vi "HTVacuum.ProcCases.vi"(0 "i ref in":refnum<vi>, 1 "selector":string, 2 "Data":T1, 3 "call cluster":T2={"Object"="", "Selector"="", "CallType"=enum."synchronous", "Async Object"="", "Async Selector"="", "Data Descriptor"="", "Data"=[], "Error #"=0, "Expire"=0}, 5 "error in (no error)":errorcluster) -> (14 "i ref out":refnum<vi>, 17 "answer cluster":T2={"Object"="", "Selector"="", "CallType"=enum."synchronous", "Async Object"="", "Async Selector"="", "Data Descriptor"="", "Data"=[], "Error #"=0, "Expire"=0}, 19 "error out":errorcluster)   [LabVIEW 2014, in "HTVacuum.lvlib"]
doc: "This method is called by a process from within the default case in the event loop. The methods of a class that are linked to events will be called from THIS method. Add your code here."
uses:
  HTVacuum.lvlib
  CS_Core/CSSystem/CoreDefs/CoreDefs.call_type.ctl
  CS_Core/BaseProcess/BaseProcess.descriptor string definition.ctl
  CS_Core/CSSystem/CoreDefs/CoreDefs.rawDataType.ctl
  CS_Core/CSSystem/CoreLib/CoreLib.string 2 byte array.vi
  CS_Core/CSSystem/CoreLib/CoreLib.short 2 byte array.vi
  CS_Core/CSSystem/CoreLib/CoreLib.byte array 2 int.vi
  CS_Core/CSSystem/CoreLib/CoreLib.int 2 byte array.vi
  CS_Core/BaseProcess/BaseProcess.lvlib
  CS_Core/CSSystem/CoreLib/CoreLib.lvlib
  CS_Core/CSApplicationBaseClasses/DeviceBase/DeviceBase.lvlib
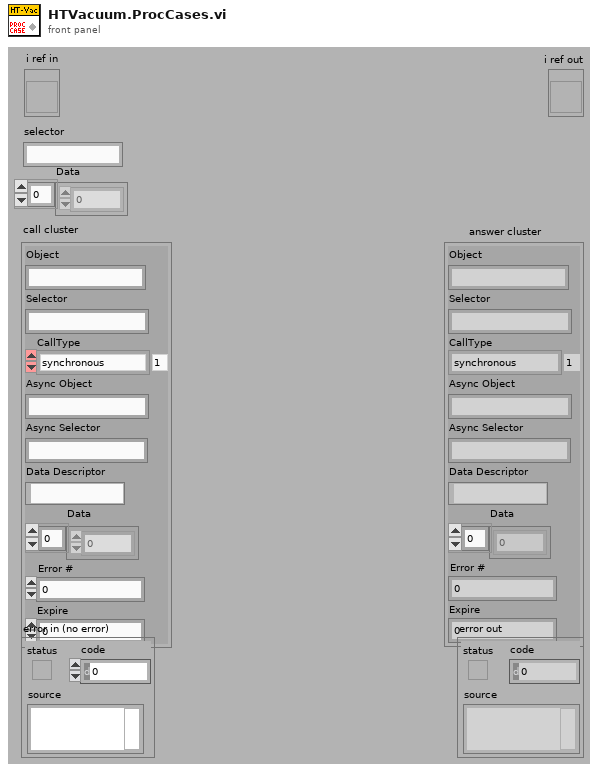
[diagram p1: front panel]
types:
  T1 = typedef "CoreDefs.rawDataType.ctl" = i8[]
  T2 = typedef "CoreDefs.call_type.ctl" = cluster{"Object":string, "Selector":string, "CallType":enum16{"simple", "synchronous", "asynchronous"}, "Async Object":string, "Async Selector":string, "Data Descriptor":T3, "Data":T1, "Error #":i32, "Expire":u32}
  T3 = typedef "BaseProcess.lvlib/BaseProcess.descriptor string definition.ctl" = string
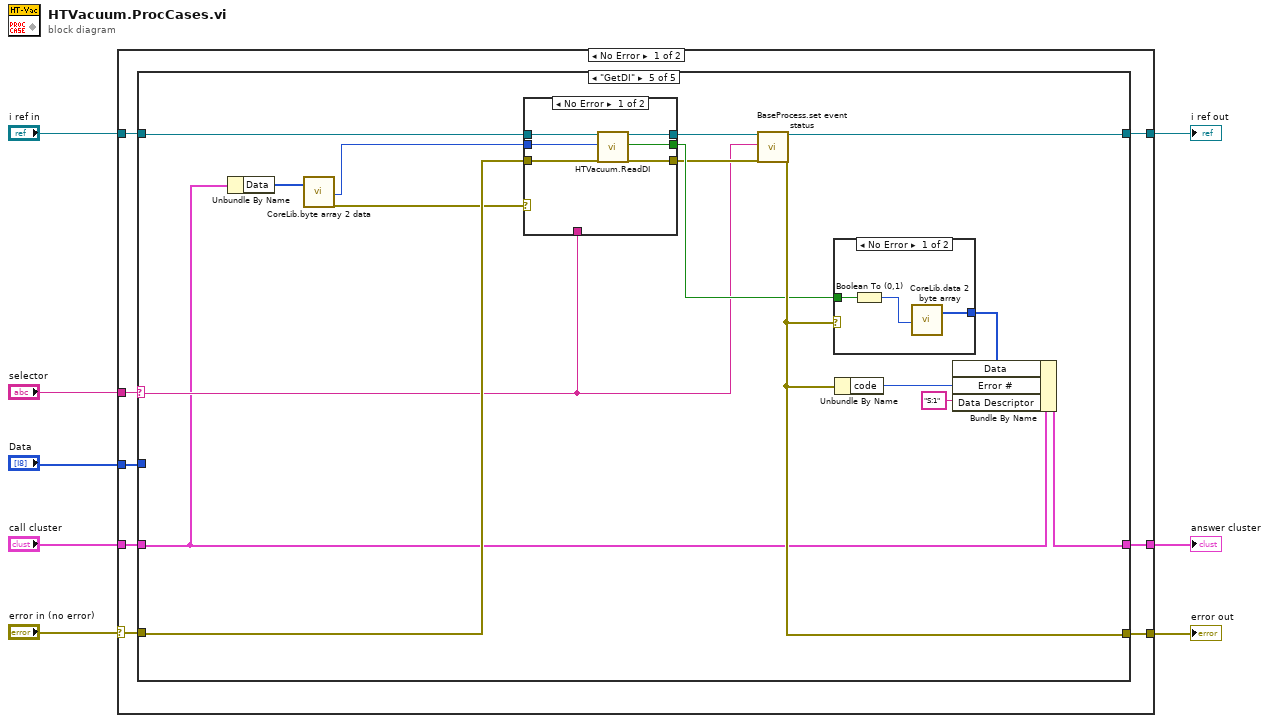
[diagram p0: block diagram]
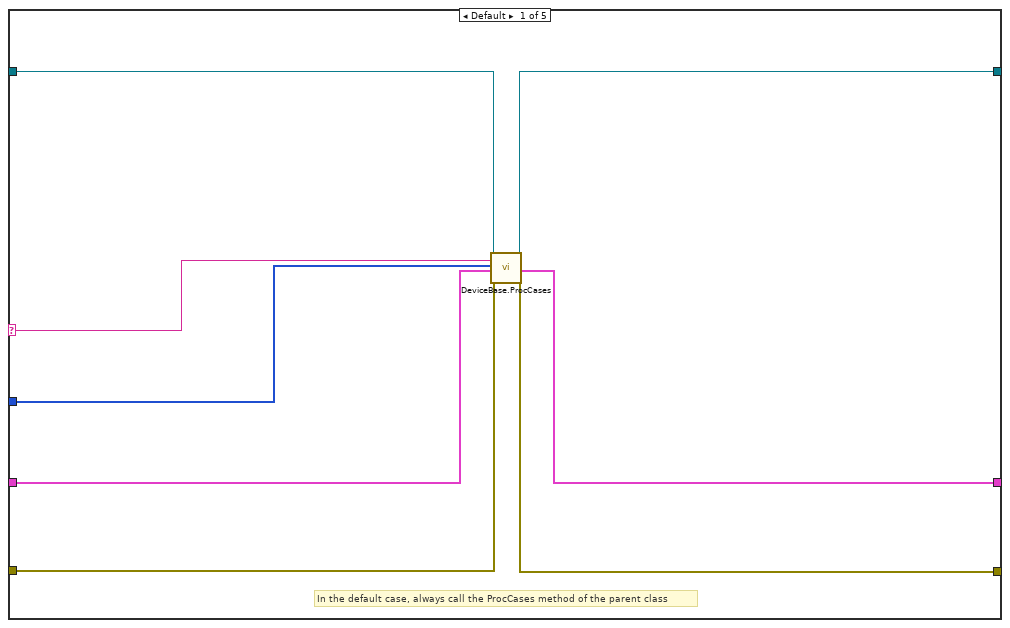
[diagram p2: hidden frame]
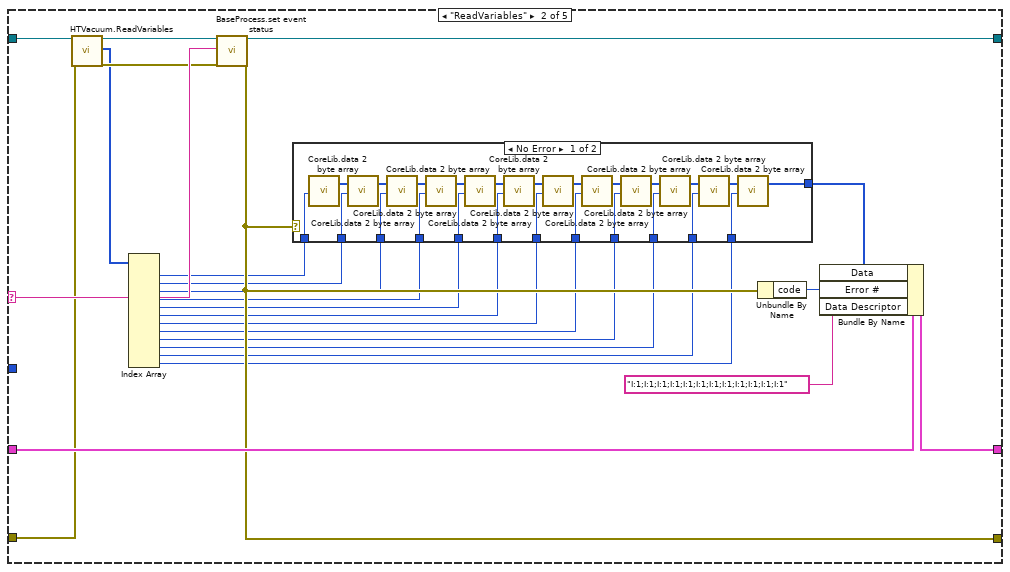
[diagram p3: hidden frame]
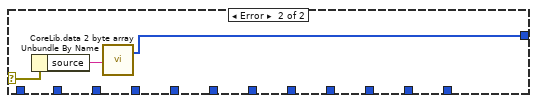
[diagram p4: hidden frame]
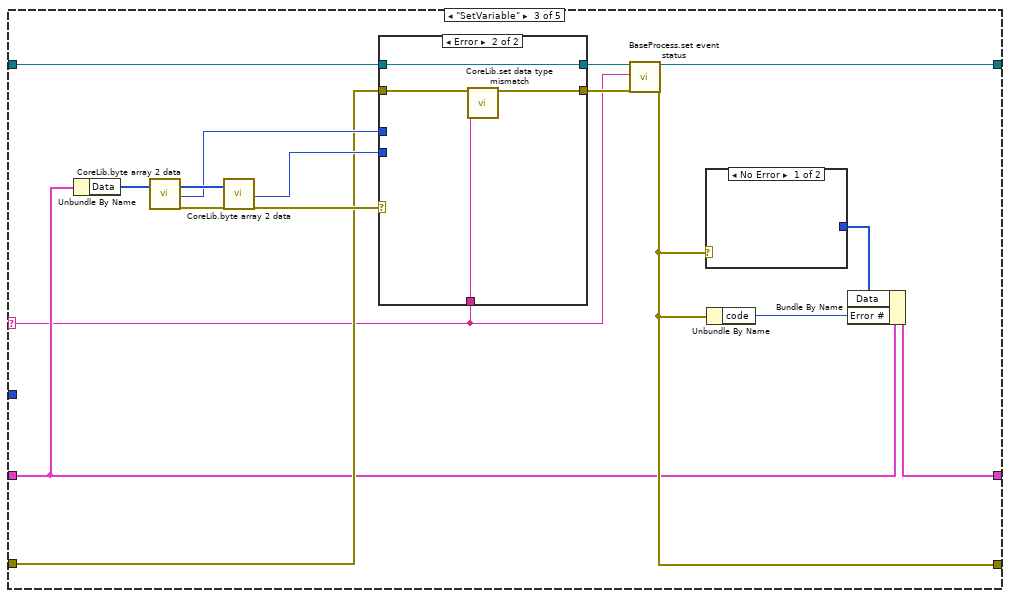
[diagram p5: hidden frame]
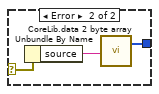
[diagram p6: hidden frame]
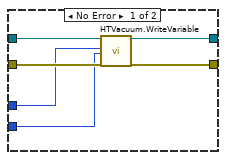
[diagram p7: hidden frame]
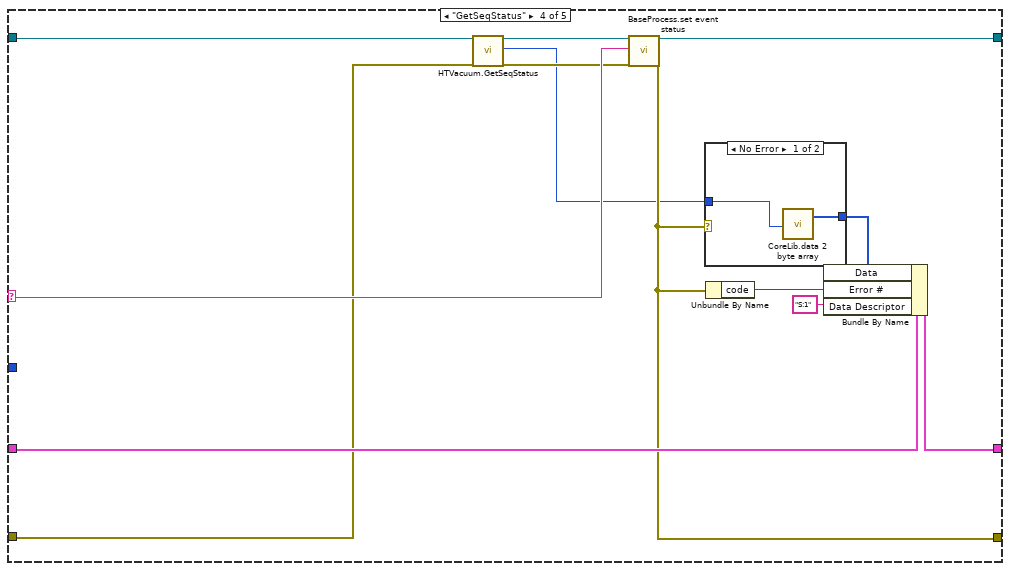
[diagram p8: hidden frame]
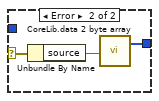
[diagram p9: hidden frame]
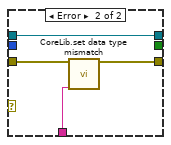
[diagram p10: hidden frame]
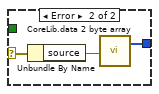
[diagram p11: hidden frame]
diagram:
  n1 = case shown="No Error" "error in (no error)" {
    selector: "error in (no error)" -> [w9 w157]
    tunnel: "selector" -> [w16 _]
    tunnel: [w15 w158] -> w7
    tunnel: "Data" -> [w14 _]
    tunnel: "call cluster" -> [w13 w158]
    tunnel: "i ref in" -> [w12 w159]
    tunnel: [w11 w159] -> w3
    tunnel: [w10 w157] -> w2
    frame No Error {
      n2 = case shown="\"GetDI\"" w16 {
        selector: w16 -> [w20 w44 w78 w115 w129]
        tunnel: w14 -> [w19 _ _ _ _]
        tunnel: w12 -> [w24 w41 w79 w111 w134]
        tunnel: [w23 w43 w77 w116 w137] -> w11
        tunnel: w13 -> [w18 w48 w80 w114 w126]
        tunnel: [w17 w47 w81 w113 w136] -> w15
        tunnel: w9 -> [w22 w38 w83 w109 w131]
        tunnel: [w21 w45 w82 w112 w135] -> w10
        frame Default {
          # "In the default case, always call the ProcCases method of the parent class"
          n3 = call "DeviceBase.ProcCases.vi"("i ref in"=w24, "selector"=w20, "Data"=w19, "call cluster"=w18, "error in (no error)"=w22) -> ("i ref out"=w23:refnum<vi>, "answer cluster"=w17:T2, "error out"=w21:errorcluster)  [unwired: 12 in]
        }
        frame "ReadVariables" {
          n4 = call "HTVacuum.ReadVariables.vi"("i ref in"=w41, "error in (no error)"=w38) -> ("i ref out"=w40:refnum<vi>, "U-VAR values"=w37:i32[], "error out"=w39:errorcluster)  [unwired: 15 in]
          n5 = Index Array(array=w37) -> (element #1=w36:i32, element #2=w35:i32, element #3=w34:i32, element #4=w33:i32, element #5=w32:i32, element #6=w31:i32, element #7=w30:i32, element #8=w29:i32, element #9=w28:i32, element #10=w27:i32, element #11=w26:i32, element #12=w25:i32)  [unwired: 12 in]
          n6 = call "BaseProcess.set event status.vi"("i ref in"=w40, "EventStatus"=w44, "error in (no error)"=w39) -> ("i ref out"=w43:refnum<vi>, "error out"=w45:errorcluster)  [unwired: 14 in, 1 out]
          n7 = case shown="No Error" w45 {
            selector: w45 -> [_ w76]
            tunnel: [w73 w75] -> w46
            tunnel: w36 -> [w61 _]
            tunnel: w35 -> [w60 _]
            tunnel: w34 -> [w59 _]
            tunnel: w33 -> [w58 _]
            tunnel: w32 -> [w57 _]
            tunnel: w31 -> [w56 _]
            tunnel: w30 -> [w55 _]
            tunnel: w29 -> [w54 _]
            tunnel: w28 -> [w53 _]
            tunnel: w27 -> [w52 _]
            tunnel: w26 -> [w51 _]
            tunnel: w25 -> [w50 _]
            frame No Error {
              n8 = call-poly "CoreLib.data 2 byte array.vi"("i32"=w61) -> ("byteArray out"=w62:T1)  [unwired: 18 in]
              n9 = call-poly "CoreLib.data 2 byte array.vi"("byteArray"=w62, "i32"=w60) -> ("byteArray out"=w63:T1)  [unwired: 17 in]
              n10 = call-poly "CoreLib.data 2 byte array.vi"("byteArray"=w63, "i32"=w59) -> ("byteArray out"=w64:T1)  [unwired: 17 in]
              n11 = call-poly "CoreLib.data 2 byte array.vi"("byteArray"=w64, "i32"=w58) -> ("byteArray out"=w65:T1)  [unwired: 17 in]
              n12 = call-poly "CoreLib.data 2 byte array.vi"("byteArray"=w65, "i32"=w57) -> ("byteArray out"=w66:T1)  [unwired: 17 in]
              n13 = call-poly "CoreLib.data 2 byte array.vi"("byteArray"=w66, "i32"=w56) -> ("byteArray out"=w67:T1)  [unwired: 17 in]
              n14 = call-poly "CoreLib.data 2 byte array.vi"("byteArray"=w67, "i32"=w55) -> ("byteArray out"=w68:T1)  [unwired: 17 in]
              n15 = call-poly "CoreLib.data 2 byte array.vi"("byteArray"=w68, "i32"=w54) -> ("byteArray out"=w69:T1)  [unwired: 17 in]
              n16 = call-poly "CoreLib.data 2 byte array.vi"("byteArray"=w69, "i32"=w53) -> ("byteArray out"=w70:T1)  [unwired: 17 in]
              n17 = call-poly "CoreLib.data 2 byte array.vi"("byteArray"=w70, "i32"=w52) -> ("byteArray out"=w71:T1)  [unwired: 17 in]
              n18 = call-poly "CoreLib.data 2 byte array.vi"("byteArray"=w71, "i32"=w51) -> ("byteArray out"=w72:T1)  [unwired: 17 in]
              n19 = call-poly "CoreLib.data 2 byte array.vi"("byteArray"=w72, "i32"=w50) -> ("byteArray out"=w73:T1)  [unwired: 17 in]
            }
            frame Error {
              n20 = Unbundle By Name(w76) -> ("source"=w74:string)
              n21 = call-poly "CoreLib.data 2 byte array.vi"("string"=w74) -> ("byteArray out"=w75:T1)  [unwired: 18 in]
            }
          }
          n22 = Unbundle By Name(w45) -> ("code"=w49:i32)
          n23 = Bundle By Name(cluster=w48, "Data"=w46, "Error #"=w49, "Data Descriptor"="I:1;I:1;I:1;I:1;I:1;I:1;I:1;I:1;I:1;I:1;I:1;I:1") -> (w47:T2)
        }
        frame "SetVariable" {
          n24 = Unbundle By Name(w80) -> ("Data"=w89:T1)
          n25 = call-poly "CoreLib.byte array 2 data.vi"("byteArray"=w89) -> ("byteArray out"=w87:T1, "i32"=w85:i32, "error out"=w88:errorcluster)  [unwired: 16 in]
          n26 = call-poly "CoreLib.byte array 2 data.vi"("byteArray"=w87, "error in (no error)"=w88) -> ("i32"=w84:i32, "error out"=w86:errorcluster)  [unwired: 15 in, 1 out]
          n27 = case shown="Error" w86 {
            tunnel: [w101 w106] -> w91
            tunnel: w79 -> [w102 w106]
            tunnel: w83 -> [w100 w105]
            tunnel: [w99 w104] -> w90
            tunnel: w84 -> [w98 _]
            tunnel: w78 -> [_ w103]
            tunnel: w85 -> [w97 _]
            frame No Error {
              n28 = call "HTVacuum.WriteVariable.vi"("i ref in"=w102, "Var# (1)"=w97, "Value"=w98, "error in (no error)"=w100) -> ("i ref out"=w101:refnum<vi>, "error out"=w99:errorcluster)  [unwired: 14 in]
            }
            frame Error {
              n29 = call "CoreLib.set data type mismatch.vi"("error in (no error)"=w105, "error source"=w103) -> ("error out"=w104:errorcluster)  [unwired: 17 in]
            }
          }
          n30 = call "BaseProcess.set event status.vi"("i ref in"=w91, "EventStatus"=w78, "error in (no error)"=w90) -> ("i ref out"=w77:refnum<vi>, "error out"=w82:errorcluster)  [unwired: 14 in, 1 out]
          n31 = case shown="No Error" w82 {
            selector: w82 -> [_ w96]
            tunnel: [_ w95] -> w92
            frame No Error {
            }
            frame Error {
              n32 = Unbundle By Name(w96) -> ("source"=w94:string)
              n33 = call-poly "CoreLib.data 2 byte array.vi"("string"=w94) -> ("byteArray out"=w95:T1)  [unwired: 18 in]
            }
          }
          n34 = Unbundle By Name(w82) -> ("code"=w93:i32)
          n35 = Bundle By Name(cluster=w80, "Data"=w92, "Error #"=w93) -> (w81:T2)
        }
        frame "GetSeqStatus" {
          n36 = call "HTVacuum.GetSeqStatus.vi"("i ref in"=w111, "error in (no error)"=w109) -> ("i ref out"=w110:refnum<vi>, "SeqStatus"=w107:u8, "error out"=w108:errorcluster)  [unwired: 15 in]
          n37 = call "BaseProcess.set event status.vi"("i ref in"=w110, "EventStatus"=w115, "error in (no error)"=w108) -> ("i ref out"=w116:refnum<vi>, "error out"=w112:errorcluster)  [unwired: 14 in, 1 out]
          n38 = case shown="No Error" w112 {
            selector: w112 -> [_ w124]
            tunnel: [w121 w122] -> w118
            tunnel: w107 -> [w120 _]
            frame No Error {
              n39 = call-poly "CoreLib.data 2 byte array.vi"("i16"=w120) -> ("byteArray out"=w121:T1)  [unwired: 18 in]
            }
            frame Error {
              n40 = Unbundle By Name(w124) -> ("source"=w123:string)
              n41 = call-poly "CoreLib.data 2 byte array.vi"("string"=w123) -> ("byteArray out"=w122:T1)  [unwired: 18 in]
            }
          }
          n42 = Unbundle By Name(w112) -> ("code"=w119:i32)
          n43 = Bundle By Name(cluster=w114, "Data"=w118, "Error #"=w119, "Data Descriptor"="S:1") -> (w113:T2)
        }
        frame "GetDI" {
          n44 = Unbundle By Name(w126) -> ("Data"=w128:T1)
          n45 = call-poly "CoreLib.byte array 2 data.vi"("byteArray"=w128) -> ("i32"=w125:i32, "error out"=w127:errorcluster)  [unwired: 16 in, 1 out]
          n46 = case shown="No Error" w127 {
            tunnel: w134 -> [w146 w147]
            tunnel: [w145 w147] -> w133
            tunnel: [w144 _] -> w132
            tunnel: w131 -> [w143 w150]
            tunnel: [w142 w149] -> w130
            tunnel: w129 -> [_ w148]
            tunnel: w125 -> [w141 _]
            frame No Error {
              n47 = call "HTVacuum.ReadDI.vi"("i ref in"=w146, "Port#"=w141, "error in (no error)"=w143) -> ("i ref out"=w145:refnum<vi>, "Port Status"=w144:bool, "error out"=w142:errorcluster)  [unwired: 14 in]
            }
            frame Error {
              n48 = call "CoreLib.set data type mismatch.vi"("error in (no error)"=w150, "error source"=w148) -> ("error out"=w149:errorcluster)  [unwired: 17 in]
            }
          }
          n49 = call "BaseProcess.set event status.vi"("i ref in"=w133, "EventStatus"=w129, "error in (no error)"=w130) -> ("i ref out"=w137:refnum<vi>, "error out"=w135:errorcluster)  [unwired: 14 in, 1 out]
          n50 = case shown="No Error" w135 {
            selector: w135 -> [_ w156]
            tunnel: [w153 w154] -> w139
            tunnel: w132 -> [w152 _]
            frame No Error {
              n51 = Boolean To (0,1)(Boolean=w152) -> (0, 1=w151:i16)
              n52 = call-poly "CoreLib.data 2 byte array.vi"("i16"=w151) -> ("byteArray out"=w153:T1)  [unwired: 18 in]
            }
            frame Error {
              n53 = Unbundle By Name(w156) -> ("source"=w155:string)
              n54 = call-poly "CoreLib.data 2 byte array.vi"("string"=w155) -> ("byteArray out"=w154:T1)  [unwired: 18 in]
            }
          }
          n55 = Unbundle By Name(w135) -> ("code"=w140:i32)
          n56 = Bundle By Name(cluster=w126, "Data"=w139, "Error #"=w140, "Data Descriptor"="S:1") -> (w136:T2)
        }
      }
    }
    frame Error {
    }
  }
  "answer cluster" <- w7
  "i ref out" <- w3
  "error out" <- w2
